vi "Que Ex-1.vi"() -> ()   [LabVIEW 2022 SP3]
panel:
  in  "stop 3":bool
  in  "stop 2":bool
  in  "stop":bool
  out "String":string
  in  "2nd Button":bool
  in  "1st buttn":bool
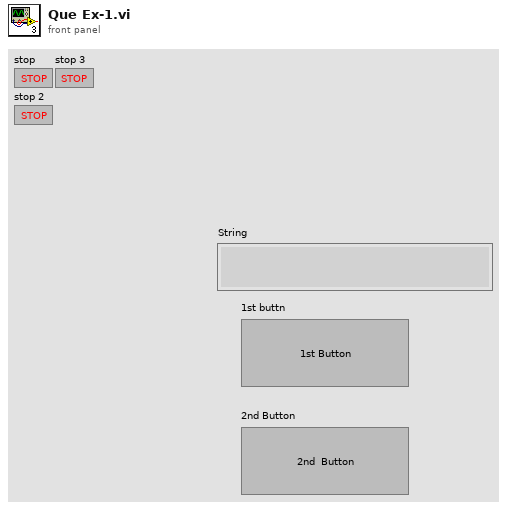
[diagram p1: front panel]
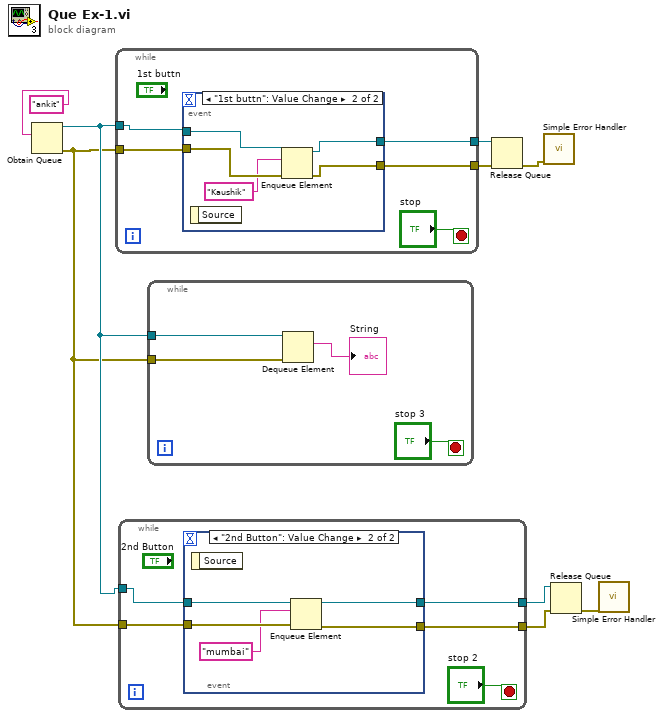
[diagram p0: block diagram]
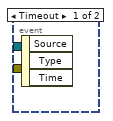
[diagram p2: hidden frame]
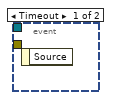
[diagram p3: hidden frame]
diagram:
  n1 = Obtain Queue(element data type="ankit") -> (queue out=w2:refnum<queue>, error out=w1:errorcluster)  [unwired: 4 in, 1 out]
  n2 = while {
    tunnel: w2 -> [w13]
    tunnel: w1 -> [w12]
    tunnel: [w11] -> w8
    tunnel: [w10] -> w7
    stop <- "stop" stop-if-true
    n3 = event shown="[1] \"1st buttn\": Value Change" {
      selector: _ -> [_ _]
      dyn-events: _ -> [_ _]
      timeout: _ -> [_ _]
      tunnel: w13 -> [_ w19]
      tunnel: w12 -> [_ w18]
      tunnel: [_ w16] -> w11
      tunnel: [_ w15] -> w10
      event Timeout {
        n4 = event-data() -> ()  [unwired: 1 in, 1 out]
      }
      event "1st buttn": Value Change {
        n5 = event-data() -> ()  [unwired: 1 in, 1 out]
        n6 = Enqueue Element(queue=w19, element="Kaushik", error in (no error)=w18) -> (queue out=w16:refnum<queue>, error out=w15:errorcluster)  [unwired: 1 in, 1 out]
      }
    }
  }
  n7 = while {
    tunnel: w2 -> [w23]
    tunnel: w1 -> [w22]
    tunnel: [w21] -> w6
    tunnel: [w20] -> w5
    stop <- "stop 2" stop-if-true
    n8 = event shown="[1] \"2nd Button\": Value Change" {
      selector: _ -> [_ _]
      dyn-events: _ -> [_ _]
      timeout: _ -> [_ _]
      tunnel: w23 -> [_ w29]
      tunnel: w22 -> [_ w28]
      tunnel: [_ w26] -> w21
      tunnel: [_ w25] -> w20
      event Timeout {
        n9 = event-data() -> ()  [unwired: 1 in, 3 out]
      }
      event "2nd Button": Value Change {
        n10 = event-data() -> ()  [unwired: 1 in, 1 out]
        n11 = Enqueue Element(queue=w29, element="mumbai", error in (no error)=w28) -> (queue out=w26:refnum<queue>, error out=w25:errorcluster)  [unwired: 1 in, 1 out]
      }
    }
  }
  n12 = while {
    tunnel: w2 -> [w32]
    tunnel: w1 -> [w31]
    stop <- "stop 3" stop-if-true
    n13 = Dequeue Element(queue=w32, error in (no error)=w31) -> (element=→"String":string)  [unwired: 1 in, 3 out]
  }
  n14 = Release Queue(queue=w8, error in (no error)=w7) -> (error out=w4:errorcluster)  [unwired: 1 in, 2 out]
  n15 = call <vilib>:"Simple Error Handler.vi"("error in (no error)"=w4) -> ()  [unwired: 4 in, 5 out]
  n16 = Release Queue(queue=w6, error in (no error)=w5) -> (error out=w3:errorcluster)  [unwired: 1 in, 2 out]
  n17 = call <vilib>:"Simple Error Handler.vi"("error in (no error)"=w3) -> ()  [unwired: 4 in, 5 out]
